vi "User Events - Fire Error Event.vi"(8 "error in":errorcluster) -> (0 "error out":errorcluster)   [LabVIEW 2024, in "User Events.lvlib"]
uses:
  User Events.lvlib
  General Type Defs/FGV States.ctl
  General Type Defs/General Type Definitions.lvlib
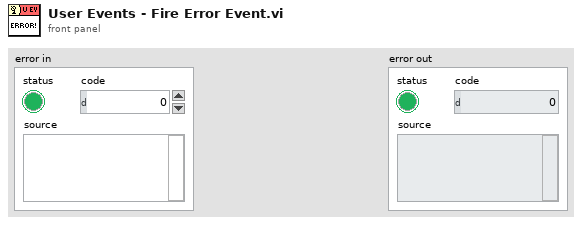
[diagram p1: front panel]
types:
  T1 = typedef "General Type Definitions.lvlib/FGV States.ctl" = enum16{"Create", "Get", "Destroy"}
  T2 = typedef "General Type Definitions.lvlib/User Events Cluster.ctl" = cluster{"STOP":refnum<user-event>, "Timeout":refnum<user-event>, "Error":refnum<user-event>}
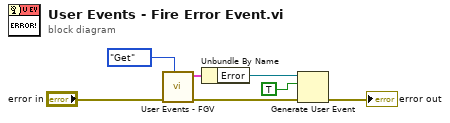
[diagram p0: block diagram]
diagram:
  n1 = call "User Events - FGV.vi"("FGV States"=FGV_States."Get", "error in"="error in") -> ("error out"=w7:errorcluster, "User Events Cluster"=w4:T2)  [unwired: 8 in]
  n2 = Unbundle By Name(w4) -> ("Error"=w5:refnum<user-event>)
  n3 = Generate User Event(user event=w5, event data cluster=TRUE ("event data"), error in=w7) -> (error out=→"error out":errorcluster)  [unwired: 1 in, 1 out]
